vi "Create.vi"(0 "object in":refnum<class "HPS-17000-PowerModule.lvclass">, 5 "configuration":string, 11 "Error In":errorcluster) -> (4 "object out":refnum<class "HPS-17000-PowerModule.lvclass">, 6 "ProcessVI Ref":refnum<vi>, 15 "Error Out":errorcluster)   [LabVIEW 2023, in "HPS-17000-PowerModule.lvlib" / "HPS-17000-PowerModule.lvclass"]
uses:
  HPS-17000-PowerModule.lvclass
  Configuration.ctl
  <vilib>/HPS-17000/Setpoint Stream Basic Config.ctl
  builds/PowerModuleInterface/PowerModuleInterface.lvlibp/Classes/PowerModule_interface/Measurements.ctl
  HPS-17000-PowerModule.lvclass/HPS-17000-PowerModule.ctl
  <vilib>/HPS-17000/Cycler.lvclass
  <vilib>/addons/_JKI.lib/Serialization/JSON/JKI JSON Serialization.lvlib
  <vilib>/Utility/LVLibp/NI_PackedLibraryUtility.lvlib
  builds/PowerModuleInterface/PowerModuleInterface.lvlibp/Classes/PowerModule_interface/PowerModuleInterface.lvclass
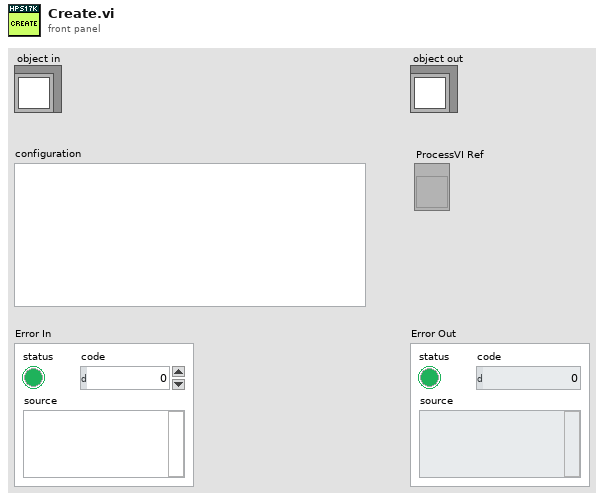
[diagram p1: front panel]
types:
  T1 = enum32{"invalid app kind", "Development System", "Run Time System", "Student Edition", "Embedded LabVIEW", "Evaluation", "Custom"}
  T2 = typedef "PowerModuleInterface.lvlibp/PowerModuleInterface.lvclass/Measurements.ctl" = cluster{"measured voltage (V)":dbl, "measured current (A)":dbl, "setpoint voltage (V)":dbl, "setpoint current (A)":dbl, "timestamp":dbl}
  T3 = enum16{"open", "replace", "create", "open or create", "replace or create", "replace or create with confirmation"}
  T4 = typedef "HPS-17000-PowerModule.lvlib/HPS-17000-PowerModule.lvclass/Configuration.ctl" = cluster{"TSN NIC IP Address":string, "HPS17000 IP Addresses":string[], "HPS Topology":enum16{"SINGLE", "MULTI"}, "Setpoint Stream Config":T5, "Measurement Array Size":i32, "Read Timeout (ms)":i32}
  T5 = typedef "Cycler.lvclass/Setpoint Stream Basic Config.ctl" = cluster{"local address":string, "receiver port":u16}
  T6 = typedef "HPS-17000-PowerModule.lvlib/HPS-17000-PowerModule.lvclass/ObjectAttributes.ctl" = cluster{"JSON Config Path":path, "Configuration":T4, "GM ID":string, "HPS17000 Refs":refnum<class "HPS-17000.lvclass">[], "connected":bool, "reserved":bool, "events":T7, "nibatterycycler_grpc_Setpoint":T8, "last timestamp":i64, "mode":T9, "range":T10, "measurement array":T2[], "measurement stream":bool, "setpoint stream":bool}
  T7 = typedef "HPS-17000.lvclass/Multi-Cycler Events.ctl" = cluster{"heartbeats events":refnum<user-event>[], "faults events":refnum<user-event>[], "network sync event":refnum<user-event>[], "setpoint status event":refnum<user-event>[]}
  T8 = typedef "NI_BC_client.lvlib/nibatterycycler_grpc_Setpoint.ctl" = cluster{"voltage":sgl, "current":sgl, "min_power":sgl, "max_power":sgl, "resistance":sgl}
  T9 = typedef "HPS-17000-PowerModule.lvlib/HPS-17000-PowerModule.lvclass/Mode.ctl" = u16
  T10 = typedef "PowerModuleInterface.lvlibp/PowerModuleInterface.lvclass/Range.ctl" = cluster{"Current Max (A)":dbl, "Current Min (A)":dbl, "Voltage Max (V)":dbl, "Voltage Min (V)":dbl}
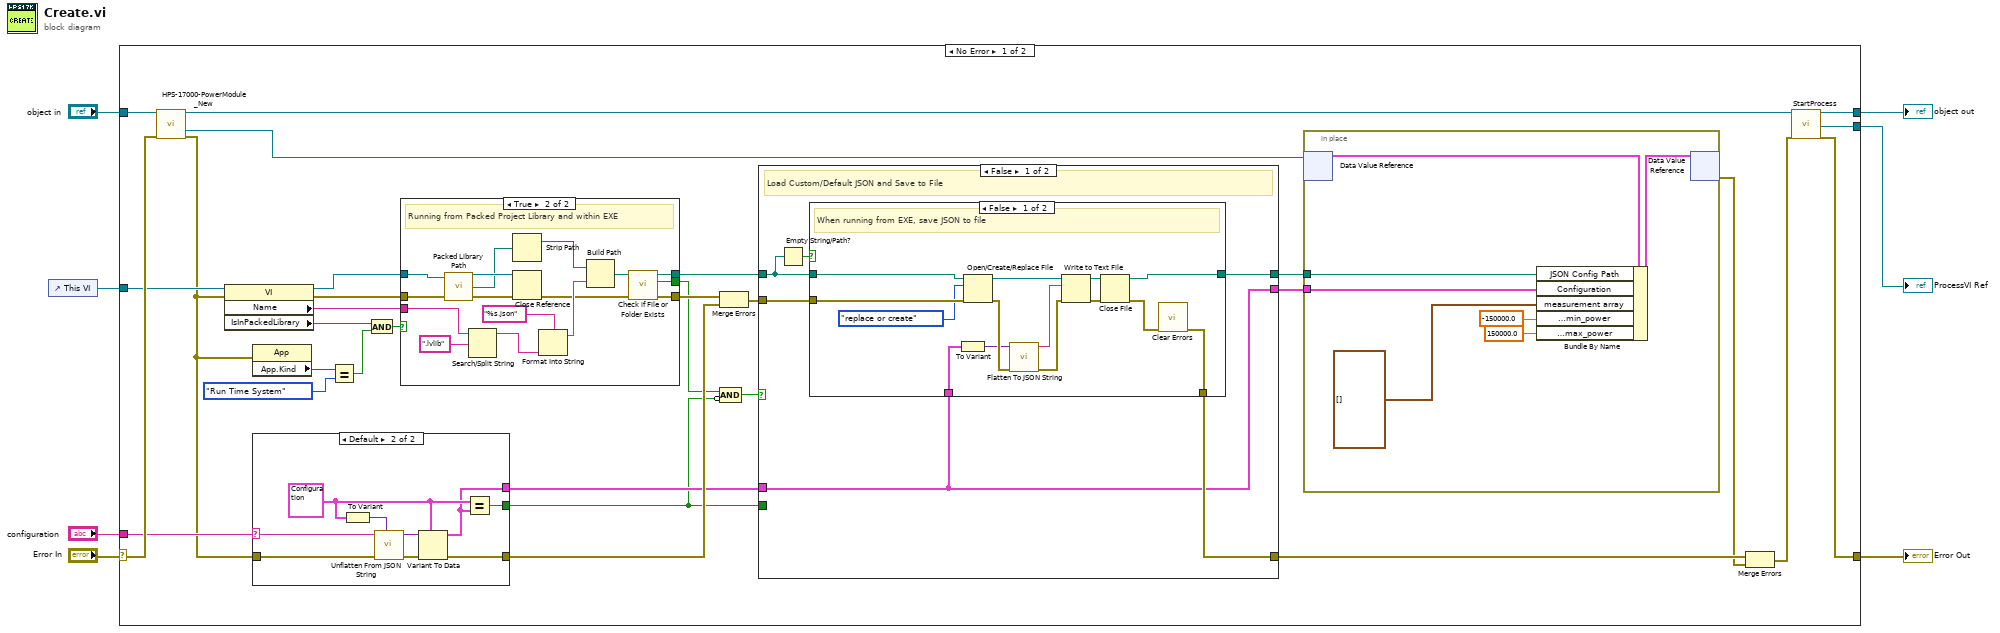
[diagram p0: block diagram]
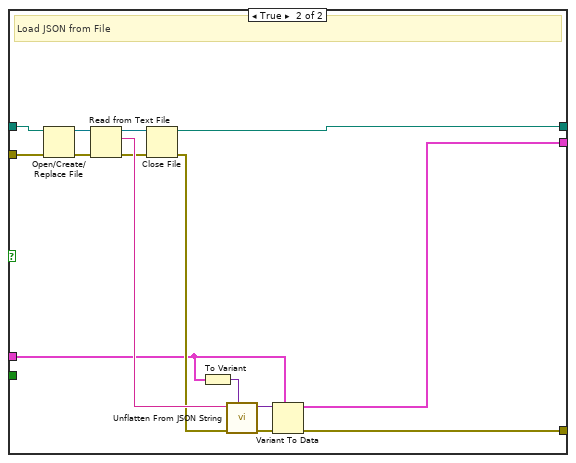
[diagram p3: hidden frame]
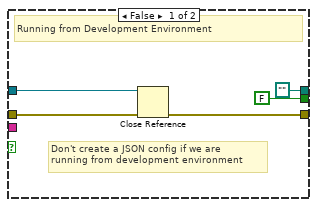
[diagram p4: hidden frame]
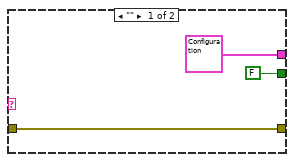
[diagram p5: hidden frame]
diagram:
  n1 = control-ref of="This VI"() -> (w1:refnum<vi>)
  n2 = case shown="No Error" "Error In" {
    selector: "Error In" -> [w37 w116]
    tunnel: "object in" -> [w38 w117]
    tunnel: "configuration" -> [w31 _]
    tunnel: [w34 w117] -> w4
    tunnel: [w33 w116] -> w3
    tunnel: [w32 _] -> w2
    tunnel: w1 -> [w30 _]
    frame No Error {
      n3 = call "HPS-17000-PowerModule_New.vi"("reference in"=w38, "Error In"=w37) -> ("reference out"=w35:refnum<class "HPS-17000-PowerModule.lvclass">, "DVRRefOut"=w36:refnum<data-value>, "Error Out"=w15:errorcluster)  [unwired: 10 in, 1 out]
      n4 = property class="VI"(reference=w30, error in=w15) -> (reference out=w28:refnum<vi>, error out=w29:errorcluster, "Name"=w16:string, "IsInPackedLibrary"=w12:bool)
      n5 = property class="App"(error in=w15) -> ("App.Kind"=w14:T1)  [unwired: 1 in, 2 out]
      n6 = case shown="Default" w31 {
        selector: w31 -> [_ w112]
        tunnel: w15 -> [w106 w115]
        tunnel: [T4 {"TSN NIC IP Address"="", "HPS17000 IP Addresses"=[], "HPS Topology"=enum."SINGLE", "Setpoint Stream Config"={"local address"="224.1.0.0", "receiver port"=61557}, "Measurement Array Size"=5000, "Read Timeout (ms)"=100} ("Configuration") w109] -> w21
        tunnel: [FALSE w108] -> w20
        tunnel: [w106 w107] -> w26
        frame "" {
        }
        frame Default {
          w110 = T4 {"TSN NIC IP Address"="", "HPS17000 IP Addresses"=[], "HPS Topology"=enum."SINGLE", "Setpoint Stream Config"={"local address"="224.1.0.0", "receiver port"=61557}, "Measurement Array Size"=5000, "Read Timeout (ms)"=100} ("Configuration")
          n7 = To Variant(anything=w110) -> (Variant=w113:variant)
          n8 = call <vilib>:"Unflatten From JSON String.vi"("Type and Defaults"=w113, "error in"=w115, "JSON String"=w112) -> ("error out"=w114:errorcluster, "Variant"=w111:variant)  [unwired: 7 in]
          n9 = Variant To Data(error in=w114, type=w110, Variant=w111) -> (data=w109:T4, error out=w107:errorcluster)
          n10 = Equal?(x=w110, y=w109) -> (x = y?=w108:bool)
        }
      }
      n11 = Equal?(x=w14, y=T1."Run Time System") -> (x = y?=w11:bool)
      n12 = And(x=w12, y=w11) -> (x .and. y?=w10:bool)
      n13 = case shown="True" w10 {
        tunnel: w29 -> [w86 w103]
        tunnel: w28 -> [w85 w102]
        tunnel: [w84 w96] -> w27
        tunnel: [FALSE ("file or folder exists?") w95] -> w24
        tunnel: [path "" w94] -> w22
        tunnel: w16 -> [_ w93]
        frame False {
          # "Don't create a JSON config if we are \nrunning from development environment"
          # "Running from Development Environment"
          n14 = Close Reference(reference=w85, error in (no error)=w86) -> (error out=w84:errorcluster)
        }
        frame True {
          # "Running from Packed Project Library and within EXE"
          n15 = call <vilib>:"Packed Library Path.vi"("error in (no error)"=w103, "vi reference"=w102) -> ("error out"=w92:errorcluster, "packed library path"=w89:path, "vi reference out"=w91:refnum<vi>)  [unwired: 1 in]
          n16 = Search/Split String(string=w93, search string/char (-)=".lvlib") -> (substring before match=w100:string)  [unwired: 1 in, 2 out]
          n17 = Strip Path(path=w89) -> (stripped path=w88:path)  [unwired: 1 out]
          n18 = Close Reference(reference=w91, error in (no error)=w92) -> (error out=w90:errorcluster)
          n19 = Format Into String(format string="%s.json", w100) -> (resulting string=w98:string)  [unwired: 2 in, 1 out]
          n20 = Build Path(base path=w88, name or relative path=w98) -> (appended path=w97:path)
          n21 = call <vilib>:"Check if File or Folder Exists.vi"("error in (no error)"=w90, "path"=w97) -> ("error out"=w96:errorcluster, "file or folder exists?"=w95:bool, "dup path"=w94:path)  [unwired: 7 in]
        }
      }
      n22 = Merge Errors(w27, w26) -> (w25:errorcluster)
      n23 = Compound Arithmetic op=AND(w24, invert w20) -> (w23:bool)
      n24 = case shown="False" w23 {
        tunnel: w25 -> [w51 w82]
        tunnel: w22 -> [w49 w81]
        tunnel: w21 -> [w46 w71]
        tunnel: w20 -> [_ _]
        tunnel: [w46 w69] -> w19
        tunnel: [w50 w70] -> w18
        tunnel: [w47 w68] -> w17
        frame False {
          # "Load Custom/Default JSON and Save to File"
          n25 = Empty String/Path?(string/path=w49) -> (empty?=w48:bool)
          n26 = case shown="False" w48 {
            tunnel: w51 -> [w62 w67]
            tunnel: [w52 w67] -> w50
            tunnel: w46 -> [w57 _]
            tunnel: w49 -> [w55 w66]
            tunnel: [w54 w66] -> w47
            frame False {
              # "When running from EXE, save JSON to file"
              n27 = To Variant(anything=w57) -> (Variant=w56:variant)
              n28 = Open/Create/Replace File(file path (use dialog)=w55, error in=w62, operation (0:open)=T3."replace or create") -> (refnum out=w65:refnum<file>, error out=w59:errorcluster)  [unwired: 3 in, 1 out]
              n29 = call <vilib>:"Flatten To JSON String.vi"("error in"=w59, "Variant"=w56) -> ("error out"=w60:errorcluster, "JSON String"=w58:string)  [unwired: 8 in]
              n30 = Write to Text File(file (use dialog)=w65, text=w58, error in=w60) -> (refnum out=w63:refnum<file>, error out=w64:errorcluster)  [unwired: 1 in, 1 out]
              n31 = Close File(refnum=w63, error in=w64) -> (path=w54:path, error out=w53:errorcluster)
              n32 = call <vilib>:"Clear Errors.vi"("error in (no error)"=w53) -> ("error out"=w52:errorcluster)  [unwired: 5 in, 1 out]
            }
            frame True {
              # "Don't save to file when running from dev environment"
            }
          }
        }
        frame True {
          # "Load JSON from File"
          n33 = Open/Create/Replace File(file path (use dialog)=w81, error in=w82) -> (refnum out=w79:refnum<file>, error out=w80:errorcluster)  [unwired: 4 in, 1 out]
          n34 = Read from Text File(file (use dialog)=w79, error in=w80) -> (refnum out=w75:refnum<file>, text=w78:string, error out=w76:errorcluster)  [unwired: 2 in, 1 out]
          n35 = Close File(refnum=w75, error in=w76) -> (path=w68:path, error out=w74:errorcluster)
          n36 = To Variant(anything=w71) -> (Variant=w77:variant)
          n37 = call <vilib>:"Unflatten From JSON String.vi"("Type and Defaults"=w77, "error in"=w74, "JSON String"=w78) -> ("error out"=w73:errorcluster, "Variant"=w72:variant)  [unwired: 7 in]
          n38 = Variant To Data(error in=w73, type=w71, Variant=w72) -> (data=w69:T4, error out=w70:errorcluster)
        }
      }
      n39 = in-place {
        in-place-border: w19 -> [w42]
        in-place-border: w17 -> [w43]
        n40 = in-place-dvr #1(w36) -> (w44:T6)  [unwired: 1 out]
        n41 = Bundle By Name(cluster=w44, "JSON Config Path"=w43, "Configuration"=w42, "measurement array"=T2[] [], "nibatterycycler_grpc_Setpoint.min_power"=sgl -150000.0, "nibatterycycler_grpc_Setpoint.max_power"=sgl 150000.0 ("nibatterycycler_grpc_Setpoint.min_power")) -> (w45:T6)
        n42 = in-place-dvr #1(w45) -> (w9:errorcluster)  [unwired: 1 out]
      }
      n43 = Merge Errors(w18, w9) -> (w8:errorcluster)
      n44 = call "StartProcess.vi"("reference in"=w35, "Error In"=w8) -> ("reference out"=w34:refnum<class "HPS-17000-PowerModule.lvclass">, "ProcessViRef"=w32:refnum<vi>, "Error Out"=w33:errorcluster)  [unwired: 13 in, 2 out]
    }
    frame Error {
    }
  }
  "Error Out" <- w3
  "object out" <- w4
  "ProcessVI Ref" <- w2
